vi "InitAnalysesVariables.vi"(9 "Ny [rows]":i32, 11 "Nx [cols]":i32) -> (3 "Stat Vars":T1)   [LabVIEW 2018]
panel:
  in  "n":i32
  in  "Ptot":dbl
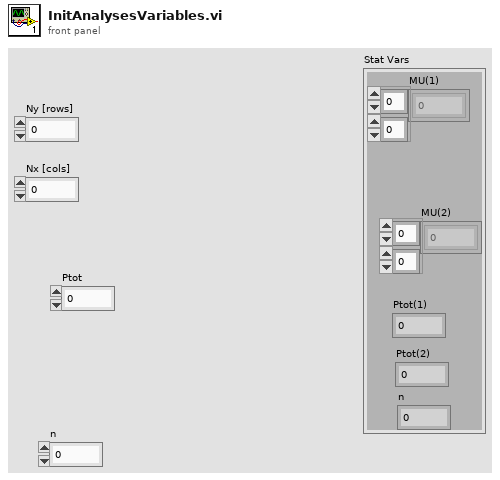
[diagram p1: front panel]
types:
  T1 = cluster{"MU(1)":dbl[][], "MU(2)":dbl[][], "Ptot(1)":dbl, "Ptot(2)":dbl, "n":i32}
  T2 = cluster{dbl[][], dbl[][], "Ptot":dbl, "Ptot":dbl, "n":i32}
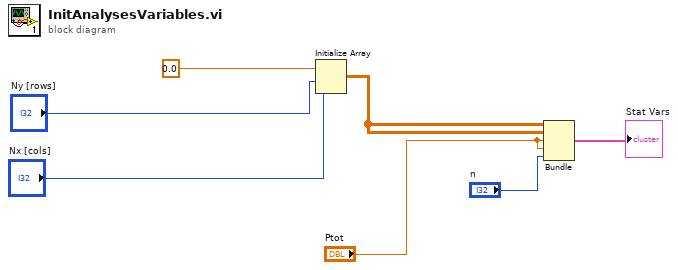
[diagram p0: block diagram]
diagram:
  n1 = Initialize Array(0.0, "Ny [rows]", "Nx [cols]") -> (w4:dbl[][])
  n2 = Bundle(w4, w4, "Ptot"="Ptot", "Ptot"="Ptot", "n"="n") -> (→"Stat Vars":T2)  [unwired: 1 in]
